vi "Parse Core.vi"(0 "Vector Path in":refnum<class "Vector 18GHz Path.lvclass">, 5 "Config Row":string[](array[string]), 11 "error in":errorcluster) -> (4 "Vector Path out":refnum<class "Vector 18GHz Path.lvclass">, 15 "error out":errorcluster)   [LabVIEW 2023, in "RFFixtureCharact.RFPM.lvlib" / "Vector 18GHz Path.lvclass"]
uses:
  Vector 18GHz Path.lvclass
  C:/rfcal/AuxTools/STSRFFixtureCharactUtility/Source/Code Modules/Common/Base Classes/Path/Path.lvclass
  Charact Result Accessor/Vector/Vector Charact Result Accessor.lvclass
  C:/rfcal/AuxTools/STSRFFixtureCharactUtility/Source/Code Modules/Fixture/RFPM/Charact Result Accessor/Base/Charact Result Accessor.lvclass
  C:/rfcal/AuxTools/STSRFFixtureCharactUtility/Source/Code Modules/Common/Result Accessor/Result Accessor.lvclass
  Common/Base Classes/Path/Path.lvclass/Path.ctl
  Common/Base Classes/Path/Properties/Read Date.vi
  Common/Base Classes/Path/Properties/Read Interval.vi
  Common/Data Cache/Settings Dictionary/Setting Keys.vi
  Public/Base Classes/Vector/Vector Abstract Path/Vector Abstract Path.lvclass
  Vector 18GHz Path.lvclass/Vector 18GHz Path.ctl
  Common/RFCalAndFixtureCharact.Common.lvlib
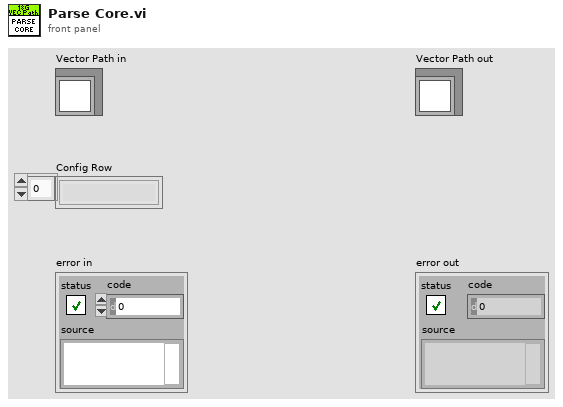
[diagram p1: front panel]
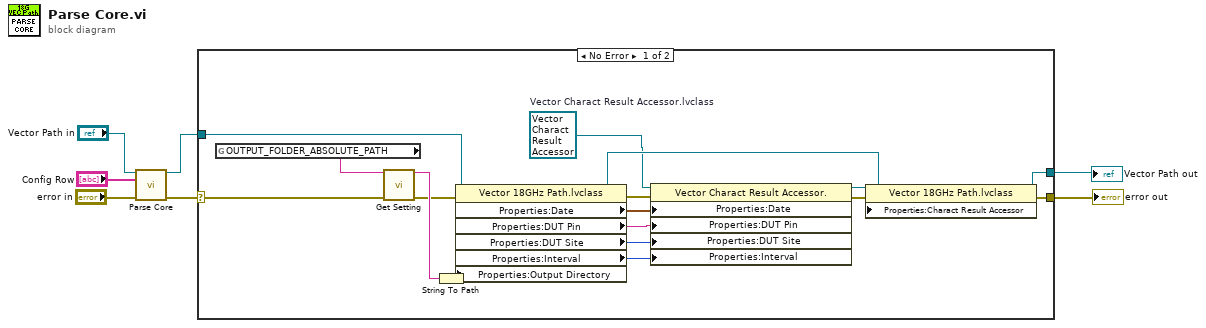
[diagram p0: block diagram]
diagram:
  n1 = call-parent "Parse Core.vi"("Vector Path in"="Vector Path in", "Config Row"="Config Row", "error in (no error)"="error in") -> ("Vector Path out"=w4:refnum<class "Vector 18GHz Path.lvclass">, "error out"=w1:errorcluster)  [unwired: 11 in]
  n2 = case shown="No Error" w1 {
    selector: w1 -> [w10 w25]
    tunnel: w4 -> [w15 w26]
    tunnel: [w14 w25] -> w3
    tunnel: [w13 w26] -> w2
    frame No Error {
      w16 = refnum<class "Vector Charact Result Accessor.lvclass"> refnum  # Vector Charact Result Accessor.lvclass
      n3 = global read "Setting Keys.vi" "OUTPUT_FOLDER_ABSOLUTE_PATH"() -> (w12:string)
      n4 = call "Get Setting.vi"("Setting name"=w12, "error in (no error)"=w10) -> ("Setting value out"=w11:string, "error out"=w9:errorcluster)  [unwired: 11 in, 1 out]
      n5 = String To Path(string=w11) -> (path=w8:path)
      n6 = property class="Vector 18GHz Path.lvclass"(reference=w15, error in=w9, "Properties:Output Directory"=w8) -> (reference out=w18:refnum<class "Vector 18GHz Path.lvclass">, error out=w23:errorcluster, "Properties:Date"=w22:timestamp, "Properties:DUT Pin"=w21:string, "Properties:DUT Site"=w20:i32, "Properties:Interval"=w19:i32)
      n7 = property class="Vector Charact Result Accessor."(reference=w16, error in=w23, "Properties:Date"=w22, "Properties:DUT Pin"=w21, "Properties:DUT Site"=w20, "Properties:Interval"=w19) -> (reference out=w17:refnum<class "Vector Charact Result Accessor.lvclass">, error out=w24:errorcluster)
      n8 = property class="Vector 18GHz Path.lvclass"(reference=w18, error in=w24, "Properties:Charact Result Accessor"=w17) -> (reference out=w13:refnum<class "Vector 18GHz Path.lvclass">, error out=w14:errorcluster)
    }
    frame Error {
    }
  }
  "error out" <- w3
  "Vector Path out" <- w2
